vi "Einheit neutral in ppm.vi"(10 "Einheit":T1, 11 "Konzentration in":dbl) -> (3 "Konzentration out":dbl)   [LabVIEW 2020, in "EPA 1065.lvlib" / "HovaCAL Interference verificaton.lvlib"]
uses:
  HovaCAL Interference verificaton.lvlib
  Linearisierung V2/SpanEinstellungen/Einheit.ctl
  Linearisierung V2/SpanEinstellungen/SpanEinstellungen.lvlib
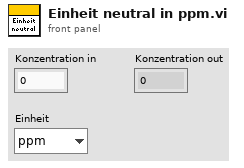
[diagram p1: front panel]
types:
  T1 = typedef "Linearisierung v2.lvlib/SpanEinstellungen.lvlib/Einheit.ctl" = enum16{"ppm", "%"}
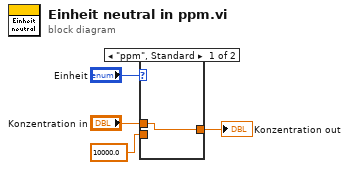
[diagram p0: block diagram]
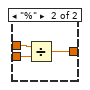
[diagram p2: hidden frame]
diagram:
  n1 = case shown="\"ppm\", Standard" "Einheit" {
    tunnel: "Konzentration in" -> [w5 w8]
    tunnel: [w5 w7] -> w4
    tunnel: 10000.0 ("y") -> [_ w6]
    frame "ppm", Default {
    }
    frame "%" {
      n2 = Divide(x=w8, y=w6) -> (x/y=w7:dbl)
    }
  }
  "Konzentration out" <- w4
